vi "Tosca-Create AI User Events.vi"() -> (4 "events":T1, 8 "Event Registration Refnum":refnum<event-registration>)   [LabVIEW 2020]
uses:
  Typedefs/Tosca-AI.ctl
  Typedefs/Tosca-AI Stream Controls.ctl
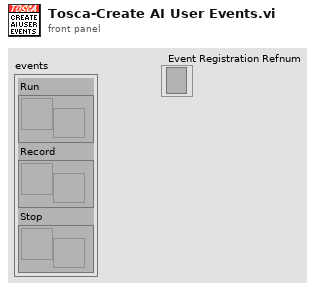
[diagram p1: front panel]
types:
  T1 = cluster{"Run":refnum<user-event>, "Record":refnum<user-event>, "Stop":refnum<user-event>}
  T2 = typedef "Tosca-AI Stream Controls.ctl" = cluster{"record":bool, "stem":string}
  T3 = typedef "Tosca-AI.ctl" = cluster{"active":bool, "Fs":dbl, "AI":string[], "DI":string[]}
  T4 = cluster{"Run":refnum<user-event>, "Stream":refnum<user-event>, "Stop":refnum<user-event>}
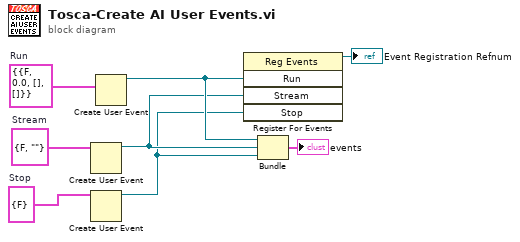
[diagram p0: block diagram]
diagram:
  w2 = T2 {"record"=FALSE, "stem"=""}  # Stream
  w5 = cluster{"exit":bool} {"exit"=FALSE}  # Stop
  w7 = cluster{"AI":T3} {"AI"={"active"=FALSE, "Fs"=0.0, "AI"=[], "DI"=[]}}  # Run
  n1 = Create User Event(user event datatype=w2) -> (user event=w6:refnum<user-event>)  [unwired: 1 in, 1 out]
  n2 = Create User Event(user event datatype=w5) -> (user event=w4:refnum<user-event>)  [unwired: 1 in, 1 out]
  n3 = Create User Event(user event datatype=w7) -> (user event=w8:refnum<user-event>)  [unwired: 1 in, 1 out]
  n4 = register-events(w8, w6, w4) -> (reference out=→"Event Registration Refnum":refnum<event-registration>)  [unwired: 2 in, 1 out]
  n5 = Bundle("Run"=w8, "Stream"=w6, "Stop"=w4) -> (→"events":T4)  [unwired: 1 in]
